vi "Defer Panel Updates.vi"(8 "error in":errorcluster, 10 "Front Panel":refnum<vi>, 11 "Defer Panel Updates":bool) -> (0 "error out":errorcluster)   [LabVIEW 2025]
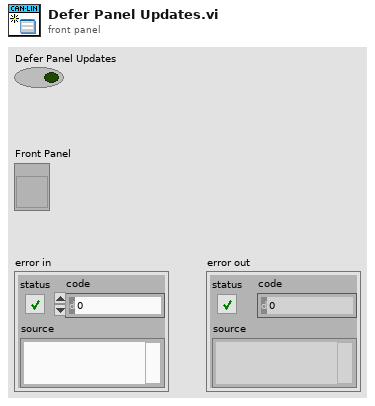
[diagram p1: front panel]
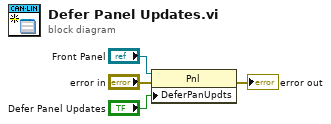
[diagram p0: block diagram]
diagram:
  n1 = property class="Pnl"(reference="Front Panel", error in="error in", "DeferPanUpdts"="Defer Panel Updates") -> (error out=→"error out":errorcluster)  [unwired: 1 out]
